vi "S2DS_DataSorting.vi"(5 "Data (in)":dbl[](array[numeric]), 7 "DAC info list":T1) -> (1 "Data (out)":dbl[](array[numeric]), 3 "DAC info list (out)":T1)   [LabVIEW 2025]
uses:
  TYPE DEFS/S2DS_DAC info new.ctl
  TYPE DEFS/S2DS_Single DC info.ctl
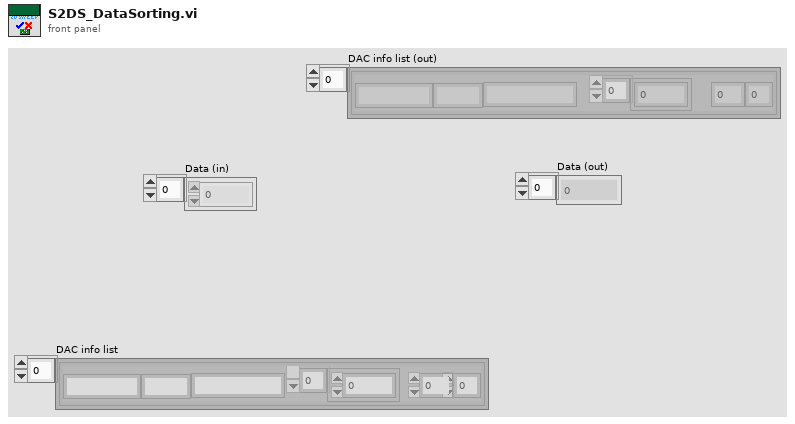
[diagram p1: front panel]
types:
  T1 = typedef "S2DS_DAC info new.ctl" = T2[]
  T2 = typedef "S2DS_Single DC info.ctl" = cluster{"Operation identifier":string, "DC parameters":dbl[], "U":i32, "V":i32, "Name":string, "Unit":string}
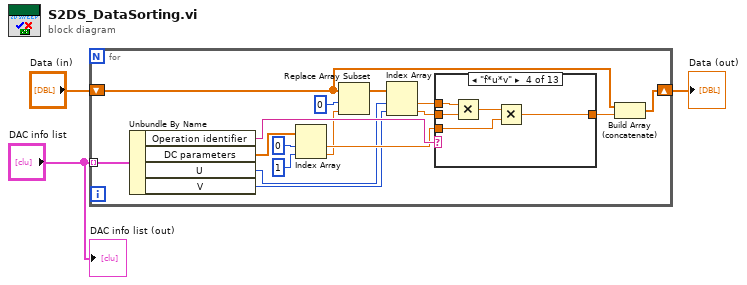
[diagram p0: block diagram]
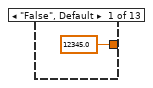
[diagram p2: hidden frame]
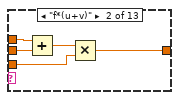
[diagram p3: hidden frame]
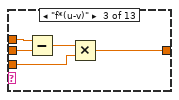
[diagram p4: hidden frame]
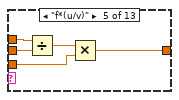
[diagram p5: hidden frame]
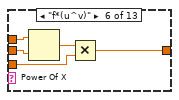
[diagram p6: hidden frame]
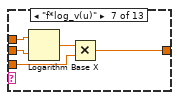
[diagram p7: hidden frame]
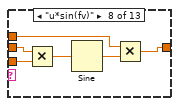
[diagram p8: hidden frame]
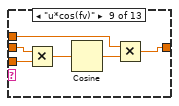
[diagram p9: hidden frame]
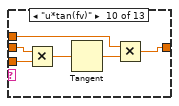
[diagram p10: hidden frame]
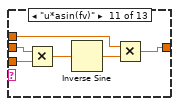
[diagram p11: hidden frame]
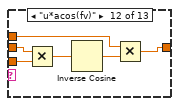
[diagram p12: hidden frame]
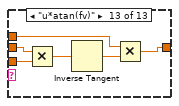
[diagram p13: hidden frame]
diagram:
  n1 = for {
    tunnel: "DAC info list" -> [w19] mode=indexing
    shift-right: [w6] -> w2
    shift-left: "Data (in)" -> [w8]
    n2 = Unbundle By Name(w19) -> ("Operation identifier"=w18:string, "DC parameters"=w14:dbl[], "U"=w5:i32, "V"=w4:i32)
    n3 = Index Array(array=w14, index #1=0 ("index"), index #2=1 ("index")) -> (element #1=w11:dbl, element #2=w10:dbl)
    n4 = Replace Array Subset(array=w8, new element=w10, index=0) -> (w9:dbl[])
    n5 = Index Array(array=w9, index #1=w5, index #2=w4) -> (element #1=w17:dbl, element #2=w16:dbl)
    n6 = case shown="\"f*u*v\"" w18 {
      tunnel: w17 -> [_ w25 w30 w35 w40 w43 w48 w53 w59 w65 w71 w77 w83]
      tunnel: w16 -> [_ w24 w29 w34 w39 w42 w47 w55 w61 w67 w73 w79 w85]
      tunnel: w11 -> [_ w22 w27 w32 w37 w45 w50 w56 w62 w68 w74 w80 w86]
      tunnel: [12345.0 w21 w26 w31 w36 w44 w49 w51 w57 w63 w69 w75 w81] -> w7
      frame "False", Default {
      }
      frame "f*(u+v)" {
        n7 = Add(x=w25, y=w24) -> (x+y=w23:dbl)
        n8 = Multiply(x=w23, y=w22) -> (x*y=w21:dbl)
      }
      frame "f*(u-v)" {
        n9 = Subtract(x=w30, y=w29) -> (x-y=w28:dbl)
        n10 = Multiply(x=w28, y=w27) -> (x*y=w26:dbl)
      }
      frame "f*u*v" {
        n11 = Multiply(x=w35, y=w34) -> (x*y=w33:dbl)
        n12 = Multiply(x=w33, y=w32) -> (x*y=w31:dbl)
      }
      frame "f*(u/v)" {
        n13 = Divide(x=w40, y=w39) -> (x/y=w38:dbl)
        n14 = Multiply(x=w38, y=w37) -> (x*y=w36:dbl)
      }
      frame "f*(u^v)" {
        n15 = Power Of X(1:w42, 2:w43) -> (0:w41:dbl)
        n16 = Multiply(x=w41, y=w45) -> (x*y=w44:dbl)
      }
      frame "f*log_v(u)" {
        n17 = Logarithm Base X(1:w47, 2:w48) -> (0:w46:dbl)
        n18 = Multiply(x=w46, y=w50) -> (x*y=w49:dbl)
      }
      frame "u*sin(fv)" {
        n19 = Multiply(x=w55, y=w56) -> (x*y=w54:dbl)
        n20 = Sine(x=w54) -> (sin(x)=w52:dbl)
        n21 = Multiply(x=w53, y=w52) -> (x*y=w51:dbl)
      }
      frame "u*cos(fv)" {
        n22 = Multiply(x=w61, y=w62) -> (x*y=w60:dbl)
        n23 = Cosine(x=w60) -> (cos(x)=w58:dbl)
        n24 = Multiply(x=w59, y=w58) -> (x*y=w57:dbl)
      }
      frame "u*tan(fv)" {
        n25 = Multiply(x=w67, y=w68) -> (x*y=w66:dbl)
        n26 = Tangent(1:w66) -> (0:w64:dbl)
        n27 = Multiply(x=w65, y=w64) -> (x*y=w63:dbl)
      }
      frame "u*asin(fv)" {
        n28 = Multiply(x=w73, y=w74) -> (x*y=w72:dbl)
        n29 = Inverse Sine(1:w72) -> (0:w70:dbl)
        n30 = Multiply(x=w71, y=w70) -> (x*y=w69:dbl)
      }
      frame "u*acos(fv)" {
        n31 = Multiply(x=w79, y=w80) -> (x*y=w78:dbl)
        n32 = Inverse Cosine(1:w78) -> (0:w76:dbl)
        n33 = Multiply(x=w77, y=w76) -> (x*y=w75:dbl)
      }
      frame "u*atan(fv)" {
        n34 = Multiply(x=w85, y=w86) -> (x*y=w84:dbl)
        n35 = Inverse Tangent(1:w84) -> (0:w82:dbl)
        n36 = Multiply(x=w83, y=w82) -> (x*y=w81:dbl)
      }
    }
    n37 = Build Array (concatenate)(w8, w7) -> (w6:dbl[])
  }
  "Data (out)" <- w2
  "DAC info list (out)" <- "DAC info list"
